vi "Rook_Init.vi"(8 "error in (no error)":errorcluster, 11 "Object in":refnum<class "Rook.lvclass">) -> (0 "error out":errorcluster, 3 "object out":refnum<class "Rook.lvclass">)   [LabVIEW 2020]
uses:
  Rook.lvclass
  C:/_repos/_personal/Chess/Chess_LV/source/Pieces/Piece.lvclass
  C:/_repos/_personal/Chess/Chess_LV/source/Pieces/Rook/Rook.lvclass
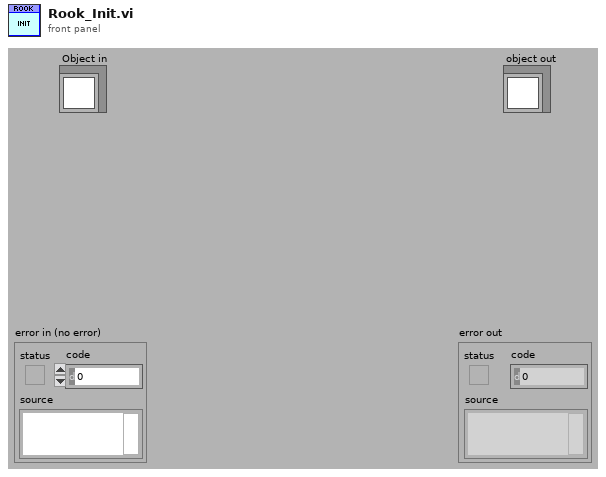
[diagram p1: front panel]
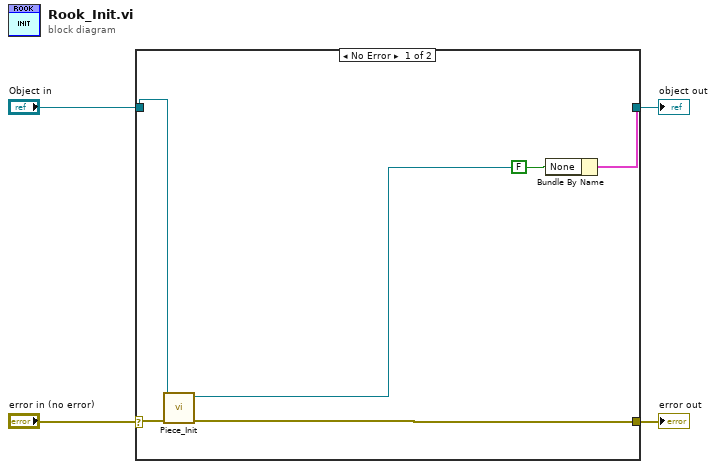
[diagram p0: block diagram]
diagram:
  n1 = case shown="No Error" "error in (no error)" {
    selector: "error in (no error)" -> [w8 w11]
    tunnel: [w10 w12] -> w4
    tunnel: "Object in" -> [w6 w12]
    tunnel: [w7 w11] -> w1
    frame No Error {
      n2 = call-dynamic "Piece_Init.vi"("error in (no error)"=w8, "object in"=w6) -> ("error out"=w7:errorcluster, "object out"=w5:refnum<class "Rook.lvclass">)  [unwired: 8 in]
      n3 = Bundle By Name(cluster=w5, "None"=FALSE) -> (w10:cluster{})
    }
    frame Error {
    }
  }
  "object out" <- w4
  "error out" <- w1
